vi "Extract List from both INI.vi"(8 "error in (no error)":errorcluster, 11 "Parameter Name":string) -> (0 "error out":errorcluster, 3 "Array":string[](array[string]))   [LabVIEW 2026, in "TALOS.lvlib"]
uses:
  TALOS.lvlib
  Ancestor/Ancestor/Ancestor.lvclass/Ancestor.ctl
  Generate Error.vi
  Circus Config Param - Core.vi
  FGV/Error Memory/Get Error Description.vi
  Get PC name.vi
  Ancestor/Ancestor/Read ID.vi
  Get Class Name.vi
  Circus Root Path.vi
  FGV/Error Memory/Error Memory Core.vi
  <vilib>/AdvancedString/Delimited String to 1D String Array.vi
  <vilib>/AdvancedString/Delimited String to 1D String Array (string).vi
  FGV/Error Memory/Error Crt Lvl checker.vi
  FGV/Error Memory/Error Memory Core.vi/40c8088d-b597-4017-91af-faa98e00292e.vi
  FGV/Error Memory/Error Memory Core.vi/d4a3ab98-063c-4e44-b43d-fbdcfe6c2be2.vi
  Global Memory.vi
  <vilib>/Utility/LVClass/Get LV Class Name.vi
  TALOS Root path.vi
  Read CSV worksheet.vi
  Global Constants.vi
  <vilib>/Utility/error.llb/General Error Handler.vi
  <vilib>/Utility/config.llb/Open Config Data.vi
  <vilib>/Utility/config.llb/Get Section Names.vi
  <vilib>/Utility/config.llb/Get Key Names.vi
  <vilib>/Utility/config.llb/Read Key.vi
  <vilib>/Utility/config.llb/Read Key (String).vi
  <vilib>/Utility/config.llb/Close Config Data.vi
  Error Log.vi
  Ancestor/Ancestor/Ancestor.lvclass
  <vilib>/Comparison/Equal/Equal Functor/Equal Functor.lvclass
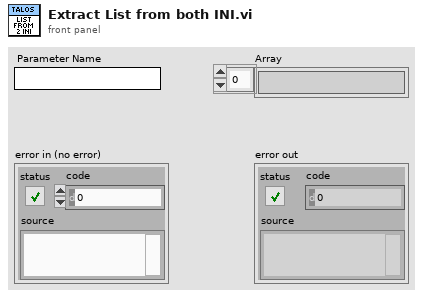
[diagram p1: front panel]
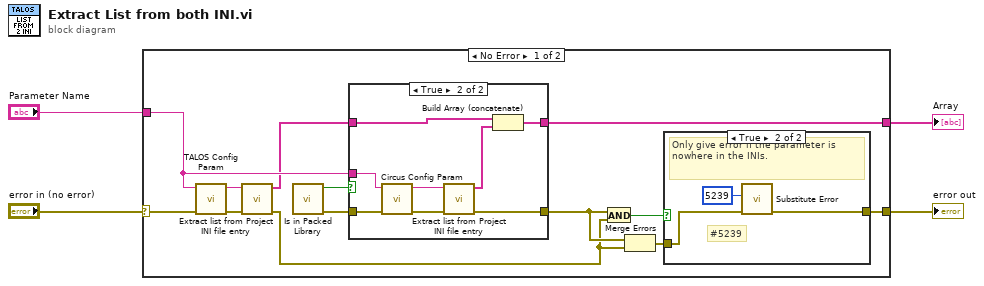
[diagram p0: block diagram]
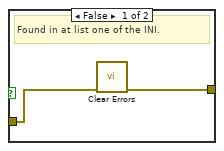
[diagram p2: hidden frame]
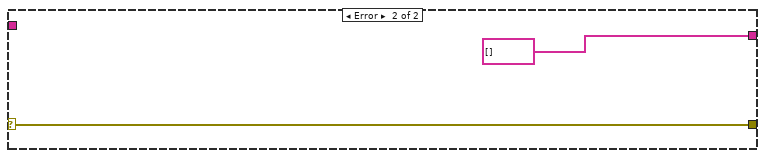
[diagram p4: hidden frame]
diagram:
  n1 = case shown="No Error" "error in (no error)" {
    selector: "error in (no error)" -> [w17 w34]
    tunnel: [w13 w34] -> w4
    tunnel: [w5 string[] []] -> w3
    tunnel: "Parameter Name" -> [w15 _]
    frame No Error {
      n2 = call "TALOS Config Param.vi"("error in (no error)"=w17, "Parameter Name"=w15) -> ("error out"=w7:errorcluster, "Output"=w9:string)  [unwired: 8 in]
      n3 = call "Extract list from Project INI file entry.vi"("error in (no error)"=w7, "Entry from INI file"=w9) -> ("error out"=w8:errorcluster, "Array"=w6:string[])  [unwired: 8 in]
      n4 = call "Is in Packed Library.vi"() -> ("error out"=w14:errorcluster, "Is In Packed Library"=w16:bool)  [unwired: 10 in]
      n5 = case shown="True" w16 {
        tunnel: w14 -> [w24 w32]
        tunnel: w15 -> [_ w31]
        tunnel: [w24 w28] -> w11
        tunnel: w6 -> [w23 w26]
        tunnel: [w23 w25] -> w5
        frame False {
        }
        frame True {
          n6 = call "Circus Config Param.vi"("error in (no error)"=w32, "Parameter Name"=w31) -> ("error out"=w29:errorcluster, "Value"=w30:string)  [unwired: 8 in]
          n7 = call "Extract list from Project INI file entry.vi"("error in (no error)"=w29, "Entry from INI file"=w30) -> ("error out"=w28:errorcluster, "Array"=w27:string[])  [unwired: 8 in]
          n8 = Build Array (concatenate)(w26, w27) -> (w25:string[])
        }
      }
      n9 = And(x=w11, y=w8) -> (x .and. y?=w12:bool)
      n10 = Merge Errors(w11, w8) -> (w10:errorcluster)
      n11 = case shown="True" w12 {
        tunnel: [w18 w22] -> w13
        tunnel: w10 -> [w19 w20]
        frame False {
          # "Found in at list one of the INI."
          n12 = call <vilib>:"Clear Errors.vi"("error in (no error)"=w19) -> ("error out"=w18:errorcluster)  [unwired: 5 in, 1 out]
        }
        frame True {
          # "#5239"
          # "Only give error if the parameter is nowhere in the INIs."
          n13 = call "Substitute Error.vi"("error in (no error)"=w20, "Error Code"=5239) -> ("error out"=w22:errorcluster)  [unwired: 9 in]
        }
      }
    }
    frame Error {
    }
  }
  "error out" <- w4
  "Array" <- w3
